vi "RVC Cartesian Motion.vi"() -> ()   [LabVIEW 2013]
uses:
  <vilib>/robotics/Kinematics/Generate Cartesian Trajectory (Int).vi
  <vilib>/robotics/Kinematics/NI_Kinematics.lvlib
panel:
  out "transformation matrix":picture
  in  "ratio":dbl(slide) scale=0.0..1.0
  in  "stop":bool
  out "Interactive Cartesian Motion":refnum<vi>(3d-picture)
  out "Cartesian Motion":refnum<vi>(3d-picture)
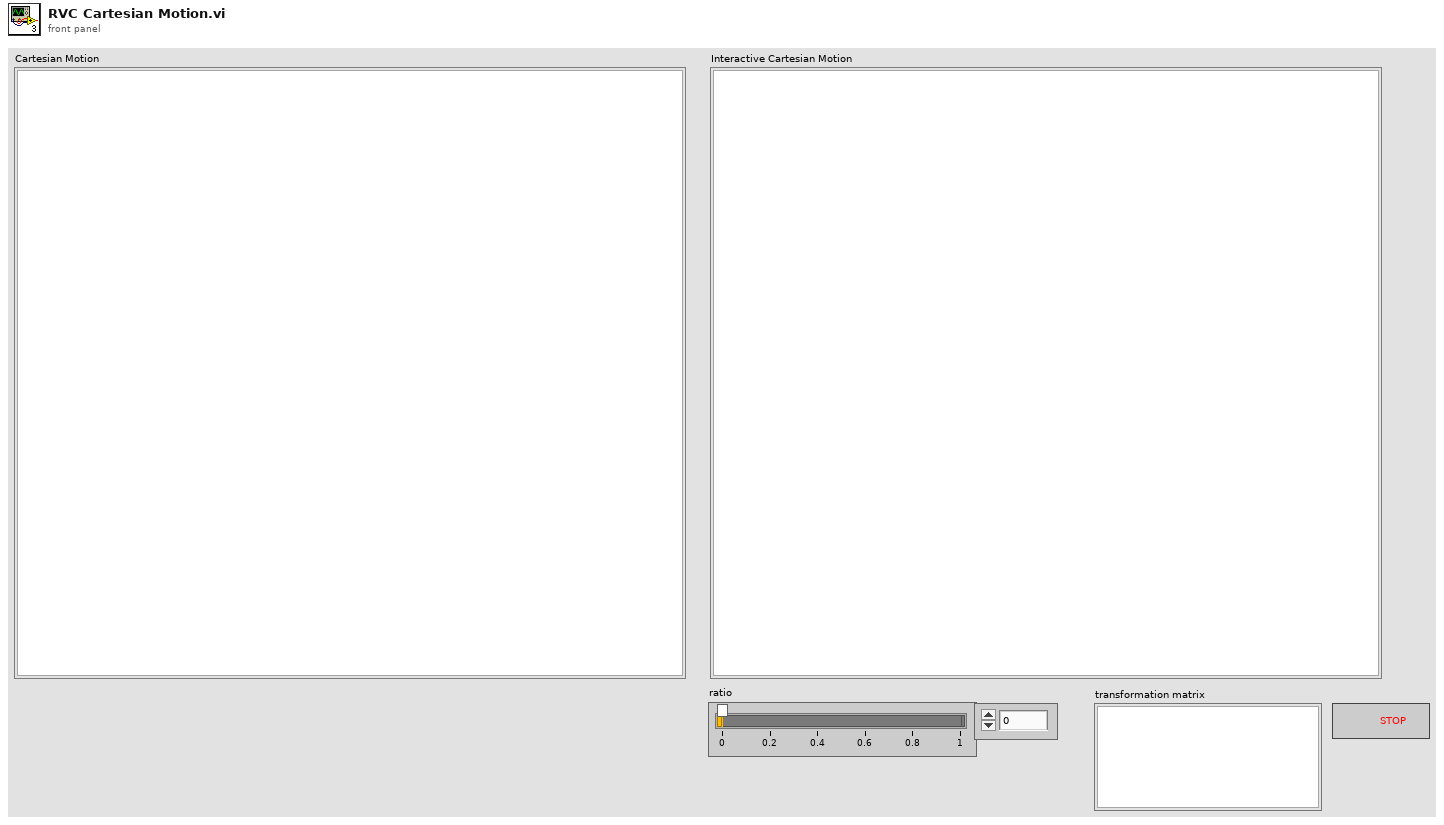
[diagram p1: front panel]
types:
  T1 = typedef "NI_Matrix.lvlib/RealMatrix.ctl" = dbl[][]
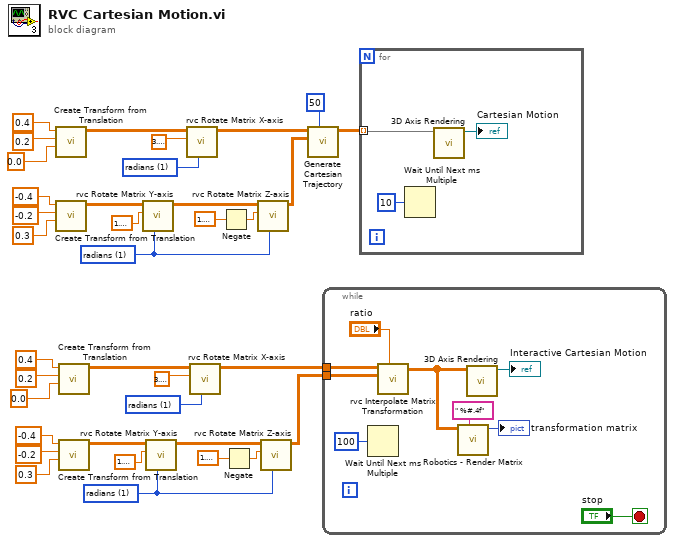
[diagram p0: block diagram]
diagram:
  w20 = u16 1 items=["degree", "radians"] ("angle unit")
  w19 = u16 1 items=["degree", "radians"] ("angle unit")
  w22 = u16 1 items=["degree", "radians"] ("angle unit")
  w23 = u16 1 items=["degree", "radians"] ("angle unit")
  n1 = call <vilib>:"Create Transform from Translation.vi"("z"=0.0 ("Numeric"), "y"=0.2 ("Numeric"), "x"=0.4 ("Numeric")) -> ("transform"=w13:T1)  [unwired: 8 in]
  n2 = call <vilib>:"Create Transform from Translation.vi"("z"=0.3 ("Numeric"), "y"=-0.2 ("Numeric"), "x"=-0.4 ("Numeric")) -> ("transform"=w15:T1)  [unwired: 8 in]
  n3 = call <vilib>:"Create Transform from Translation.vi"("z"=0.0 ("Numeric"), "y"=0.2 ("Numeric"), "x"=0.4 ("Numeric")) -> ("transform"=w28:T1)  [unwired: 8 in]
  n4 = call <vilib>:"Create Transform from Translation.vi"("z"=0.3 ("Numeric"), "y"=-0.2 ("Numeric"), "x"=-0.4 ("Numeric")) -> ("transform"=w27:T1)  [unwired: 8 in]
  n5 = call "rvc Rotate Matrix Y-axis.vi"("angle unit"=w20, "angle"=1.5707963267948966, "rotation matrix in"=w15) -> ("rotation matrix"=w18:T1)  [unwired: 8 in]
  n6 = call "rvc Rotate Matrix Y-axis.vi"("angle unit"=w22, "angle"=1.5707963267948966, "rotation matrix in"=w27) -> ("rotation matrix"=w24:T1)  [unwired: 8 in]
  n7 = call "rvc Rotate Matrix X-axis.vi"("angle unit"=w19, "angle"=3.141592653589793, "rotation matrix in"=w13) -> ("rotation matrix"=w14:T1)  [unwired: 8 in]
  n8 = call "rvc Rotate Matrix X-axis.vi"("angle unit"=w23, "angle"=3.141592653589793, "rotation matrix in"=w28) -> ("rotation matrix"=w2:T1)  [unwired: 8 in]
  n9 = Negate(x=1.5707963267948966) -> (-x=w17:dbl)
  n10 = Negate(x=1.5707963267948966) -> (-x=w25:dbl)
  n11 = call "rvc Rotate Matrix Z-axis.vi"("angle unit"=w20, "angle"=w17, "rotation matrix in"=w18) -> ("rotation matrix"=w21:T1)  [unwired: 8 in]
  n12 = call "rvc Rotate Matrix Z-axis.vi"("angle unit"=w22, "angle"=w25, "rotation matrix in"=w24) -> ("rotation matrix"=w1:T1)  [unwired: 8 in]
  n13 = call-poly <vilib>:"Generate Cartesian Trajectory.vi"("intermediate points"=50, "end transform"=w21, "start transform"=w14) -> ("interpolated trajectory"=w11:dbl[][][])  [unwired: 7 in, 1 out]
  n14 = while {
    tunnel: w2 -> [w44]
    tunnel: w1 -> [w43]
    stop <- "stop" stop-if-true
    n15 = Wait Until Next ms Multiple(millisecond multiple=u32 100) -> ()  [unwired: 1 out]
    n16 = call "rvc Interpolate Matrix Transformation.vi"("ratio"="ratio", "final transformation"=w43, "initial transformation"=w44) -> ("interpolated matrix"=w37:T1)  [unwired: 8 in]
    n17 = call "Robotics - Render Matrix.vi"("format string"=" %#.4f", "A"=w37) -> ("picture out"=→"transformation matrix":picture)  [unwired: 9 in]
    n18 = call "3D Axis Rendering.vi"("rotation matrix"=w37) -> ("SceneNode out"=→"Interactive Cartesian Motion":refnum<vi>)  [unwired: 10 in]
  }
  n19 = for {
    tunnel: w11 -> [w47] mode=indexing
    n20 = Wait Until Next ms Multiple(millisecond multiple=u32 10) -> ()  [unwired: 1 out]
    n21 = call "3D Axis Rendering.vi"("rotation matrix"=w47) -> ("SceneNode out"=→"Cartesian Motion":refnum<vi>)  [unwired: 10 in]
  }
